vi "countOccurences.vi"(10 "modifiedPaths":string[](array[string])) -> (2 "frequencyXmodifiedPaths":string[](array[string]))   [LabVIEW 2021]
uses:
  bf589c1d-03c1-744a-adca-fc2bf4ee6734.vi
  <vilib>/Comparison/Less/Less Functor/Less Functor.lvclass
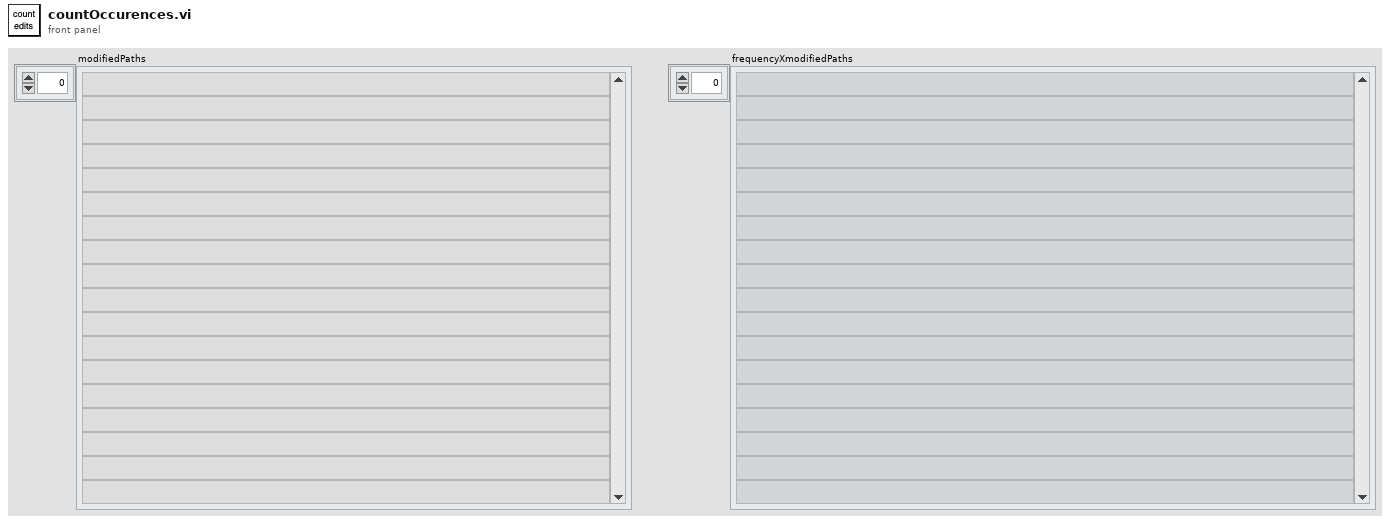
[diagram p1: front panel]
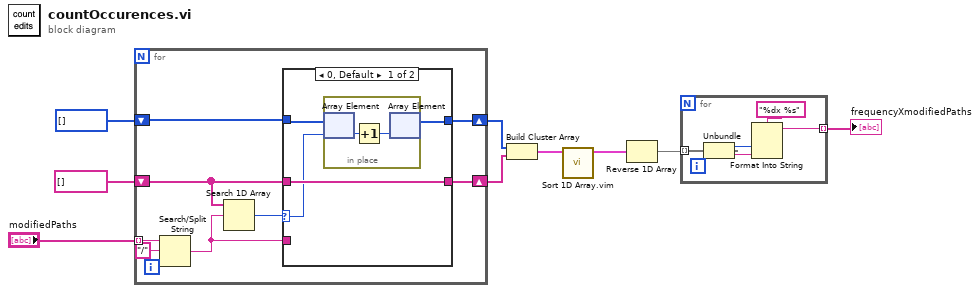
[diagram p0: block diagram]
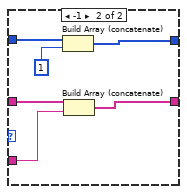
[diagram p2: hidden frame]
diagram:
  n1 = for {
    shift-right: [w15] -> w2
    shift-left: string[] [] -> [w16]
    tunnel: "modifiedPaths" -> [w12] mode=indexing
    shift-right: [w13] -> w4
    shift-left: i32[] [] -> [w14]
    n2 = Search/Split String(string=w12, search string/char (-)="/") -> (match + rest of string=w10:string)  [unwired: 1 in, 2 out]
    n3 = Search 1D Array(1D array=w16, element=w10) -> (index of element=w17:i32)  [unwired: 1 in]
    n4 = case shown="0, Default" w17 {
      selector: w17 -> [w19 _]
      tunnel: w10 -> [_ w29]
      tunnel: w16 -> [w21 w28]
      tunnel: [w21 w27] -> w15
      tunnel: w14 -> [w20 w26]
      tunnel: [w18 w25] -> w13
      frame 0, Default {
        n5 = in-place {
          n6 = in-place-array #1(w20, w19) -> (w23:i32)
          n7 = Increment(x=w23) -> (x+1=w22:i32)
          n8 = in-place-array #1(w22) -> (w18:i32[])  [unwired: 1 out]
        }
      }
      frame -1 {
        n9 = Build Array (concatenate)(w26, 1) -> (w25:i32[])
        n10 = Build Array (concatenate)(w28, w29) -> (w27:string[])
      }
    }
  }
  n11 = Build Cluster Array(w4, w2) -> (w6:cluster{i32, "relevantPath":string}[])
  n12 = call "Sort 1D Array.vim"("unsorted array"=w6) -> ("sorted array"=w5:cluster{i32, "relevantPath":string}[])  [unwired: 10 in]
  n13 = Reverse 1D Array(array=w5) -> (reversed array=w3:cluster{i32, "relevantPath":string}[])
  n14 = for {
    tunnel: w3 -> [w34] mode=indexing
    tunnel: [w30] -> w1 mode=indexing
    n15 = Unbundle(w34) -> (w33:i32, "relevantPath"=w32:string)
    n16 = Format Into String(format string="%dx %s", w33, w32) -> (resulting string=w30:string)  [unwired: 2 in, 1 out]
  }
  "frequencyXmodifiedPaths" <- w1
